vi "Power Meter.vi"(8 "error in (no error)":errorcluster, 11 "Power Meter in":refnum<class "Power Meter.lvclass">) -> (0 "error out":errorcluster, 3 "Power Meter out":refnum<class "Power Meter.lvclass">)   [LabVIEW 2009, in "Power Meter.lvclass"]
uses:
  Power Meter.lvclass
  Global/GPIB Numbers.vi
panel:
  out "Status":string
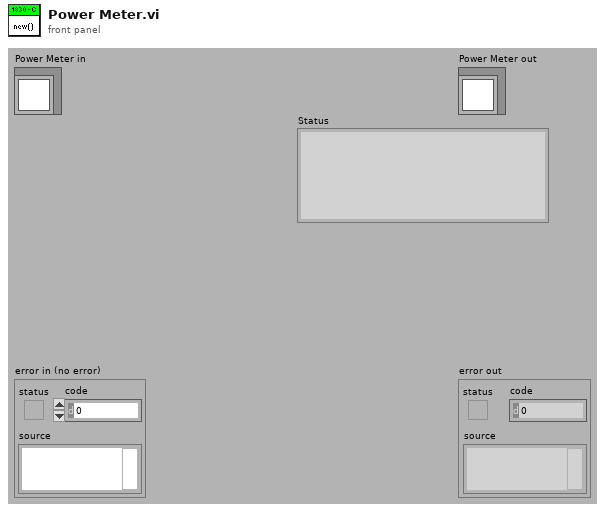
[diagram p1: front panel]
types:
  T1 = typedef "GPIB Type Def.ctl" = cluster{"Name":string, "bus":dbl, "GPIB":dbl, "GPIB as string":string, "byte":i32, "VISA Resource Name":refnum<visa-resource-name>}
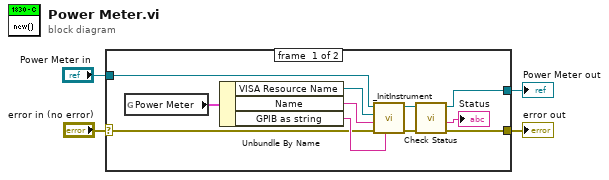
[diagram p0: block diagram]
diagram:
  n1 = case shown="No Error" "error in (no error)" {
    selector: "error in (no error)" -> [w5 w17]
    tunnel: [w7 w17] -> w3
    tunnel: [w12 w16] -> w1
    tunnel: "Power Meter in" -> [w11 w16]
    frame #0 {
      n2 = global read "GPIB Numbers.vi" "Power Meter"() -> (w15:T1)
      n3 = Unbundle By Name(w15) -> ("VISA Resource Name"=w10:refnum<visa-resource-name>, "Name"=w6:string, "GPIB as string"=w9:string)
      n4 = call-dynamic "_InitInstrument.vi"("GPIB as string"=w9, "error in (no error)"=w5, "Name"=w6, "VISA Resource Name"=w10, "Instrument in"=w11) -> ("error out"=w8:errorcluster, "Instrument out"=w14:refnum<class "Power Meter.lvclass">)  [unwired: 1 in, 4 out]
      n5 = call-dynamic "Check Status.vi"("error in (no error)"=w8, "Power Meter in"=w14) -> ("error out"=w7:errorcluster, "Status"=→"Status":string, "Power Meter out"=w12:refnum<class "Power Meter.lvclass">)  [unwired: 6 in, 1 out]
    }
    frame #1 {
    }
  }
  "error out" <- w3
  "Power Meter out" <- w1
